vi "Calibrate Ticks 2 Acceleration (uSMC).vi"(1 "Acceleration (ticks)":u8) -> (0 "Acceleration (ms)":u16)   [LabVIEW 2010, in "SignalWriterMH110203USBStepperMotor.lvclass"]
uses:
  SignalWriterMH110203USBStepperMotor.lvclass
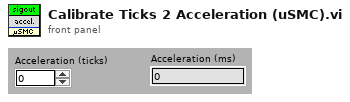
[diagram p1: front panel]
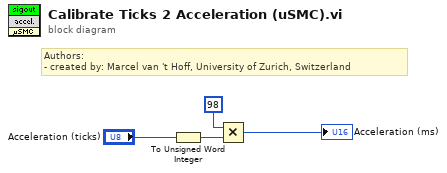
[diagram p0: block diagram]
diagram:
  # "Authors: \n- created by: Marcel van 't Hoff, University of Zurich, Switzerland"
  n1 = To Unsigned Word Integer(number="Acceleration (ticks)") -> (unsigned 16bit integer=w3:u16)
  n2 = Multiply(x=u16 98, y=w3) -> (x*y=→"Acceleration (ms)":u16)
